vi "2asumofnnatural.vi"() -> ()   [LabVIEW 2013]
panel:
  out "output":dbl
  in  "constant":dbl
  in  "input":dbl
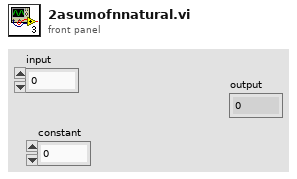
[diagram p1: front panel]
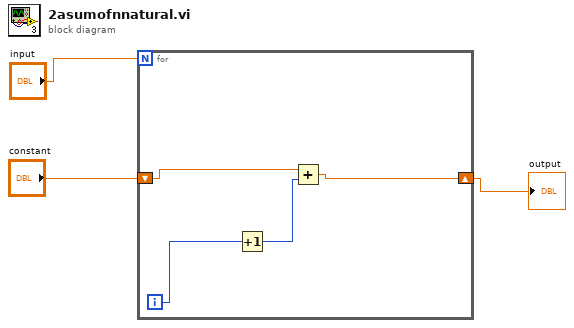
[diagram p0: block diagram]
diagram:
  n1 = for {
    N: "input" -> [_]
    shift-right: [w4] -> w1
    shift-left: "constant" -> [w7]
    i -> [w6]
    n2 = Increment(x=w6) -> (x+1=w5:i32)
    n3 = Add(x=w7, y=w5) -> (x+y=w4:dbl)
  }
  "output" <- w1
